vi "Menu_LV Class Control.vi"(11 "Affected Items Out":T1) -> (3 "Menu Items To Add":T2(array[cluster]))   [LabVIEW 2023]
uses:
  top/BundleMagic.ctl
  controls/action enum.ctl
panel:
  out "Enabled Status":enum8{"Enabled", "Disabled"}[](array[ring])
  out "Menu Item Display Name":string[](array[string])
  out "Position In Menu":T3(array[cluster])
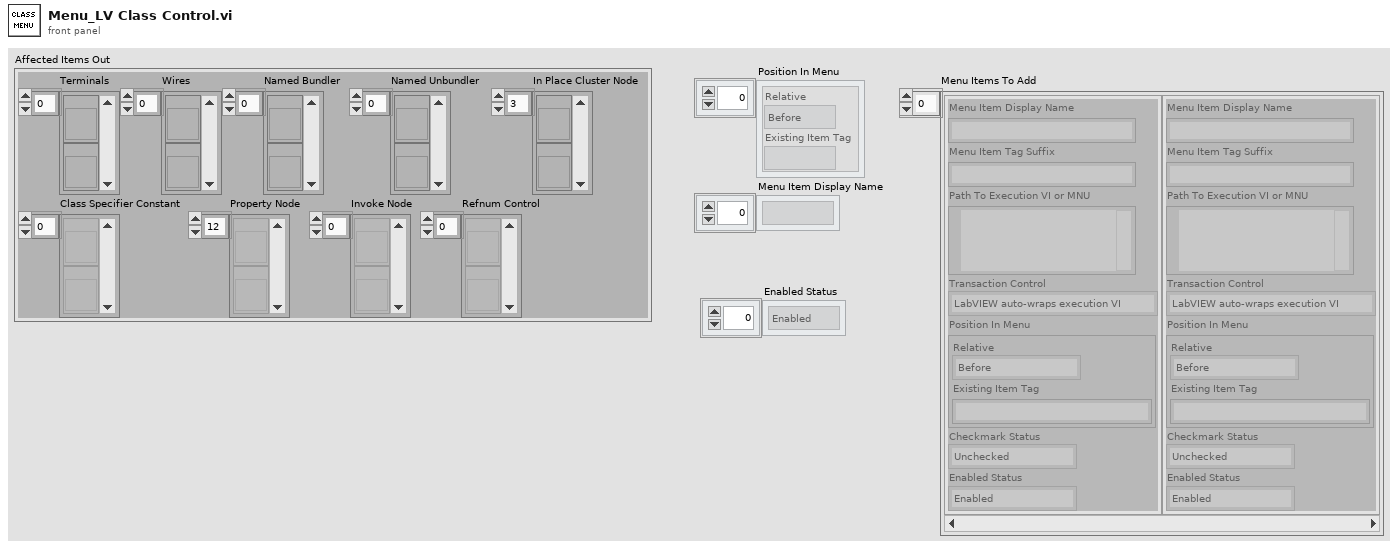
[diagram p1: front panel]
types:
  T1 = typedef "BundleMagic.ctl" = cluster{"Terminals":refnum<vi>[], "Wires":refnum<vi>[], "Named Bundler":refnum<vi>[], "Named Unbundler":refnum<vi>[], "In Place Cluster Node":refnum<vi>[], "Class Specifier Constant":refnum<vi>[], "Property Node":refnum<vi>[], "Invoke Node":refnum<vi>[], "Refnum Control":refnum<vi>[]}
  T2 = cluster{"Menu Item Display Name":string, "Menu Item Tag Suffix":string, "Path To Execution VI or MNU":path, "Transaction Control":enum8{"LabVIEW auto-wraps execution VI", "Execution VI will define if needed"}, "Position In Menu":cluster{"Relative":enum8{"Before", "Instead of", "After", "Into Submenu"}, "Existing Item Tag":string}, "Checkmark Status":enum8{"Unchecked", "Checked"}, "Enabled Status":enum8{"Enabled", "Disabled"}}[]
  T3 = cluster{"Relative":enum8{"Before", "Instead of", "After", "Into Submenu"}, "Existing Item Tag":string}[]
  T4 = typedef "action enum.ctl" = enum16{"[NONE]", "APP_SEPARATOR", "Wire Bundle", "Wire Unbundle", "Terminal Unbundle", "Terminal Bundle", "Bundler Move Up", "Bundler Move Down", "Bundler Insert", "Bundler Remove", "Bundler Remove Unwired", "Bundler Rearrange", "In Place Insert", "In Place Remove", "In Place Remove Unwired", "In Place Rearrange", "Wire Properties", "Wire Method", "Terminal Properties", "Terminal Method", "Property Move Up", "Property Move Down", "Properties Insert", "Properties Remove", "Properties Remove Unwired", "Properties Rearrange", "Method Change", "Class For Constant", "Class For Control", "Class For Node", "Class Name to Clipboard"}
  T5 = cluster{"Menu Item Display Name":string, "Menu Item Tag Suffix":string, "Path To Execution VI or MNU":path, "Transaction Control":enum8{"LabVIEW auto-wraps execution VI", "Execution VI will define if needed"}, "Position In Menu":cluster{"Relative":enum8{"Before", "Instead of", "After", "Into Submenu"}, "Existing Item Tag":string}, "Checkmark Status":enum8{"Unchecked", "Checked"}, "Enabled Status":enum8{"Enabled", "Disabled"}}
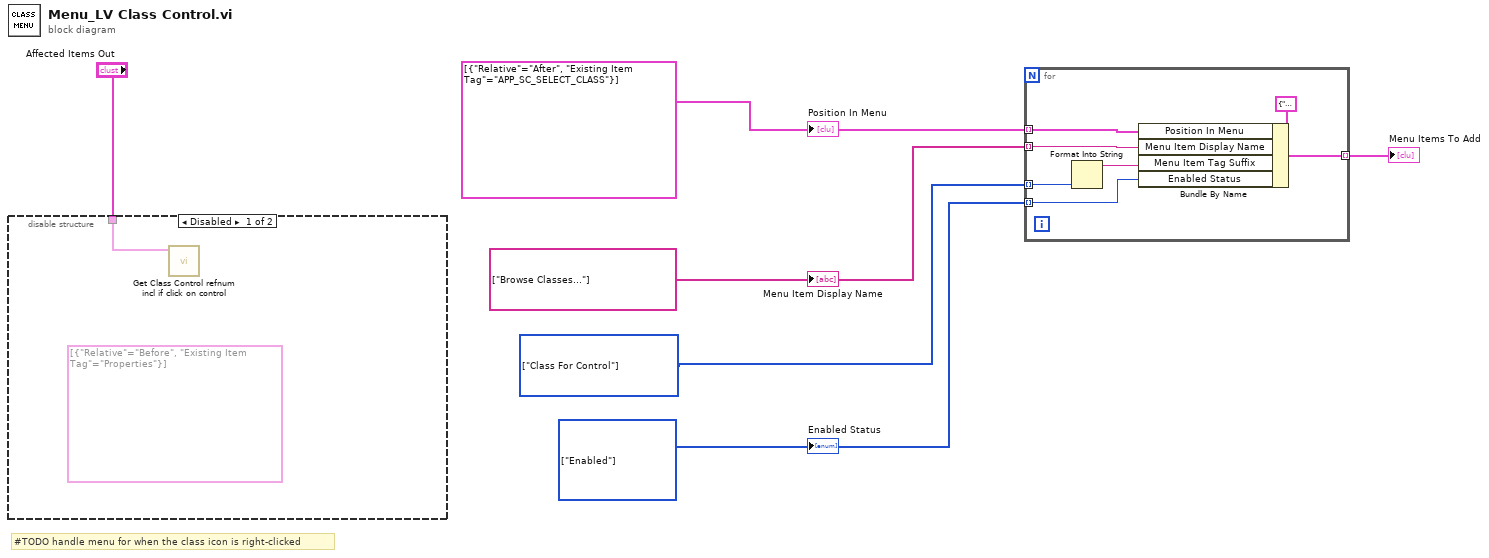
[diagram p0: block diagram]
diagram:
  w1 = T4[] [enum."Class For Control"] items=["[NONE]", "APP_SEPARATOR", "Wire Bundle", "Wire Unbundle", "Terminal Unbundle", "Terminal Bundle", "Bundler Move Up", "Bundler Move Down", "Bundler Insert", "Bundler Remove", "Bundler Remove Unwired", "Bundler Rearrange", "In Place Insert", "In Place Remove", "In Place Remove Unwired", "In Place Rearrange", "Wire Properties", "Wire Method", "Terminal Properties", "Terminal Method", "Property Move Up", "Property Move Down", "Properties Insert", "Properties Remove", "Properties Remove Unwired", "Properties Rearrange", "Method Change", "Class For Constant", "Class For Control", "Class For Node", "Class Name to Clipboard"] ("Array")
  w6 = T3 [{"Relative"=enum."After", "Existing Item Tag"="APP_SC_SELECT_CLASS"}]
  w4 = enum8{"Enabled", "Disabled"}[] [enum."Enabled"] items=["Enabled", "Disabled"]
  w5 = string[] ["Browse Classes..."]
  # "#TODO handle menu for when the class icon is right-clicked"
  n1 = disable-structure shown="Disabled" {
    disable-tunnel: "Affected Items Out" -> [w7 _]
    frame Disabled {
      (unwired) T3 [{"Relative"=enum."Before", "Existing Item Tag"="Properties"}]
      n2 = call "Get Class Control refnum incl if click on control.vi"("Affected Items"=w7) -> ()  [unwired: 9 in, 2 out]
    }
    frame Enabled {
    }
  }
  n3 = for {
    tunnel: [w14] -> w3 mode=indexing
    tunnel: w5 -> [w13] mode=indexing
    tunnel: w1 -> [w8] mode=indexing
    tunnel: w6 -> [w11] mode=indexing
    tunnel: w4 -> [w10] mode=indexing
    n4 = Format Into String(w8) -> (resulting string=w9:string)  [unwired: 3 in, 1 out]
    n5 = Bundle By Name(cluster=T5 {"Menu Item Display Name"="", "Menu Item Tag Suffix"="", "Path To Execution VI or MNU"=path "", "Transaction Control"=enum."LabVIEW auto-wraps execution VI", "Position In Menu"={"Relative"=enum."Before", "Existing Item Tag"=""}, "Checkmark Status"=enum."Unchecked", "Enabled Status"=enum."Enabled"} ("Cluster"), "Position In Menu"=w11, "Menu Item Display Name"=w13, "Menu Item Tag Suffix"=w9, "Enabled Status"=w10) -> (w14:T5)
  }
  "Menu Items To Add" <- w3
  "Position In Menu" <- w6
  "Menu Item Display Name" <- w5
  "Enabled Status" <- w4
